vi "Scratchpad.vi"() -> ()   [LabVIEW 2022 SP3, in "Conditum-Example.lvlib"]
uses:
  Conditum-Example.lvlib
  Conditum/Entity Manager/Entity Manager.lvclass
  Conditum/Database Platform/Database Platform.lvclass
  Conditum/Entity Repository/Entity Repository.lvclass
  Conditum/Entity/Entity.lvclass
  Conditum/Result Row/Result Row.lvclass
panel:
  out "Array":cluster{"String":string, u8}[](array[cluster]) {"?" format="%02x"}
  in  "String":string
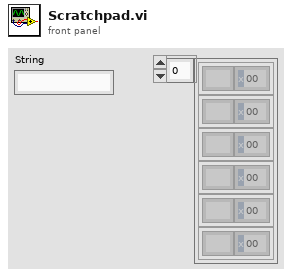
[diagram p1: front panel]
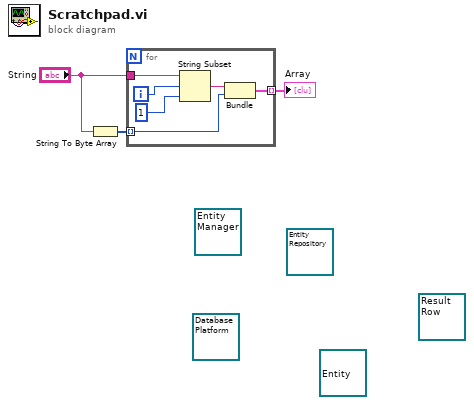
[diagram p0: block diagram]
diagram:
  (unwired) refnum<class "Result Row.lvclass"> refnum ("Conditum:Result Row")
  (unwired) refnum<class "Entity.lvclass"> refnum ("Conditum:Entity")
  (unwired) refnum<class "Entity Repository.lvclass"> refnum ("Conditum:Entity Repository")
  (unwired) refnum<class "Database Platform.lvclass"> refnum ("Conditum:Database")
  (unwired) refnum<class "Entity Manager.lvclass"> refnum ("Conditum:Entity Manager")
  n1 = String To Byte Array(string="String") -> (unsigned byte array=w2:u8[])
  n2 = for {
    tunnel: "String" -> [w9]
    tunnel: w2 -> [w5] mode=indexing
    tunnel: [w4] -> w1 mode=indexing
    i -> [w8]
    n3 = String Subset(string=w9, offset (0)=w8, length (rest)=1 ("length (rest)")) -> (substring=w6:string)
    n4 = Bundle("String"=w6, w5) -> (w4:cluster{"String":string, u8})  [unwired: 1 in]
  }
  "Array" <- w1
